vi "DrawTextBox_Create.vi"(10 "error in":errorcluster, 11 "document":refnum<k24>) -> (2 "error out":errorcluster, 3 "DrawTextBox":refnum<k24>)   [LabVIEW 2009]
uses:
  C:/Projets/LAVAG/OpenOfficeRGT/AODL/DLLs/AODL.dll
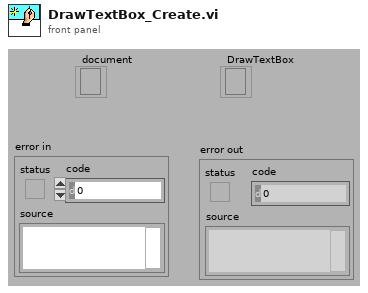
[diagram p1: front panel]
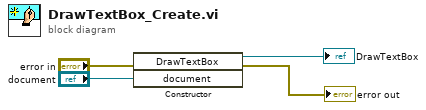
[diagram p0: block diagram]
diagram:
  n1 = constructor class="DrawTextBox"(error in="error in", "document"="document") -> (reference out=→"DrawTextBox":refnum<k24>, error out=→"error out":errorcluster)  [unwired: 2 in, 2 out]
